vi "Add.vi"(10 "Element":T1, 11 "TypedCircularBuffer in":refnum<class "LogCircularBuffer.lvclass">) -> (1 "overflow?":bool, 2 "overflow element":T1, 3 "TypedCircularBuffer out":refnum<class "LogCircularBuffer.lvclass">)   [LabVIEW 2024, in "LogCircularBuffer.lvclass"]
uses:
  LogCircularBuffer.lvclass
  Type.ctl
  RQMHCore/ErrorReporting/Record/LogRecord.lvclass
  LogCircularBuffer.lvclass/LogCircularBuffer.ctl
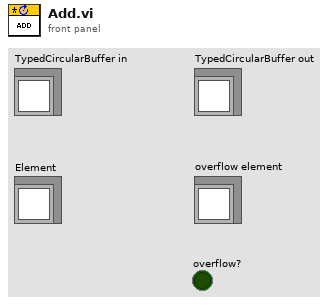
[diagram p1: front panel]
types:
  T1 = typedef "LogCircularBuffer.lvclass/Type.ctl" = refnum<class "LogRecord.lvclass">
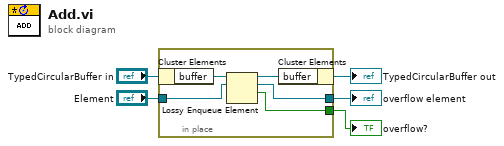
[diagram p0: block diagram]
diagram:
  n1 = in-place {
    in-place-border: "Element" -> [w9]
    in-place-border: [w8] -> w3
    in-place-border: [w7] -> w2
    n2 = in-place-cluster #1("TypedCircularBuffer in") -> ("buffer"=w10:refnum<queue>)
    n3 = Lossy Enqueue Element(queue=w10, element=w9) -> (queue out=w6:refnum<queue>, overflow element=w8:T1, overflow?=w7:bool)  [unwired: 1 in, 1 out]
    n4 = in-place-cluster #1("buffer"=w6) -> (→"TypedCircularBuffer out":refnum<class "LogCircularBuffer.lvclass">)
  }
  "overflow element" <- w3
  "overflow?" <- w2
